vi "Tip Withdraw_MFP3D.vi"() -> ()   [LabVIEW 2019]
doc: "This VI withdraw the tip. (Basically close the Z loop)."
panel:
  out "error out":errorcluster
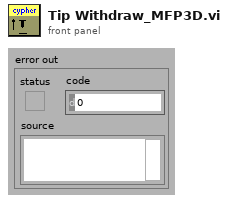
[diagram p1: front panel]
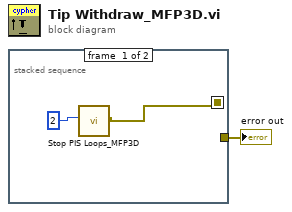
[diagram p0: block diagram]
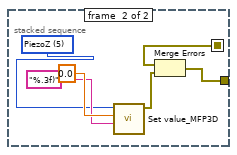
[diagram p2: hidden frame]
diagram:
  n1 = stacked-sequence {
    seq-local: [w2 _] -> [_ w9]
    tunnel: [_ w8] -> w1
    frame #0 {
      n2 = call "Stop PIS Loops_MFP3D.vi"("PIS Loop Number (0-5)"=u32 2) -> ("error out"=w2:errorcluster)  [unwired: 10 out]
    }
    frame #1 {
      w5 = u16 5 items=["OutA_52kHz", "OutB_52kHz", "OutC_78Hz", "PiezoX", "PiezoY", "PiezoZ", "DDS_Frequency1", "DDS_Frequency2", "DDS_Amplitude1", "DDS_Amplitude2"] ("Output")
      n3 = call "Set value_MFP3D.vi"("Number resolutio"="%.3f)", "Value"=0.0, "Output"=w5) -> ("error out"=w4:errorcluster)  [unwired: 8 in]
      n4 = Merge Errors(w9, w4) -> (w8:errorcluster)
    }
  }
  "error out" <- w1
